vi "Encode COB-ID.vi"(1 "Function code":T1=12 items=["EMCY"=1, "PDO1 (tx)"=3, "PDO1 (rx)"=4, "PDO2 (tx)"=5, "PDO2 (rx)"=6, "PDO3 (tx)"=7, "PDO3 (rx)"=8, "PDO4 (tx)"=9, "PDO4 (rx)"=10, "SDO (tx)"=11, "SDO (rx)"=12, "NMT error control"=14], 2 "Node-ID":u8) -> (0 "COD-ID":u32 format="%.0x")   [LabVIEW 2026, in "canopen_.lvlib" / "CANopen.lvclass"]
doc: "Computes the canonical COB-ID given the function code and the node ID. The implementation follows the algorithm described in CiA draft standard 301, page 78."
uses:
  CANopen.lvclass
  CANopen.lvclass/CANopen.ctl
  FunctionCode.ctl
  CANopen Master.lvlib
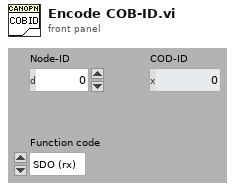
[diagram p1: front panel]
types:
  T1 = typedef "CANopen Master.lvlib/FunctionCode.ctl" = u16
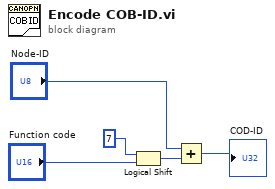
[diagram p0: block diagram]
diagram:
  n1 = Logical Shift(y=i16 7, x="Function code") -> (x << y=w4:T1)
  n2 = Add(x="Node-ID", y=w4) -> (x+y=→"COD-ID":T1)
